vi "DLPVA-100-B_&_F_Set.vi"(6 "Filter":bool=TRUE, 8 "AC/DC":bool=TRUE, 9 "Gain_2 i":bool, 10 "Gain_1 i":bool, 11 "Index":i32) -> (0 "Overload":bool, 1 "Gain_2 o":bool, 2 "Gain_1o":bool, 3 "Gain (dB)":dbl)   [LabVIEW 2013]
uses:
  driver/Control/Set_Bandwidth_DLPVA-Series.vi
  driver/Control/Set_Gain_DLPVA-100-B&F_Series.vi
  driver/FEMTO_LUCI-10.lvlib
panel:
  out "Gain_Stages 2":bool[](array[boolean])=[FALSE, FALSE, FALSE, TRUE, FALSE, FALSE, FALSE, FALSE, FALSE, FALSE, FALSE, FALSE, FALSE, FALSE, FALSE, FALSE, FALSE, FALSE, FALSE, FALSE, FALSE, FALSE, FALSE, FALSE, FALSE, FALSE, FALSE, FALSE, FALSE, FALSE, FALSE, FALSE]
  # "Remote Control LUCI-10 DLPVA-100"
  # "DLPVA-100-B & F"
  # "Configuration"
  # "Gain Setting"
  # "Overal Gain"
  # "80 dB"
  # "60 dB"
  # "Device Information"
  # "40 dB"
  # "20 dB"
  # "Filter"
  # "Coupling"
  # "Sophisticated Tools for Signal Recovery"
  # "AC"
  # "DC"
  # "1 kHz"
  # "100 kHz"
  # "20 dB"
  # "40 dB"
  # "0 dB"
  # "0 dB"
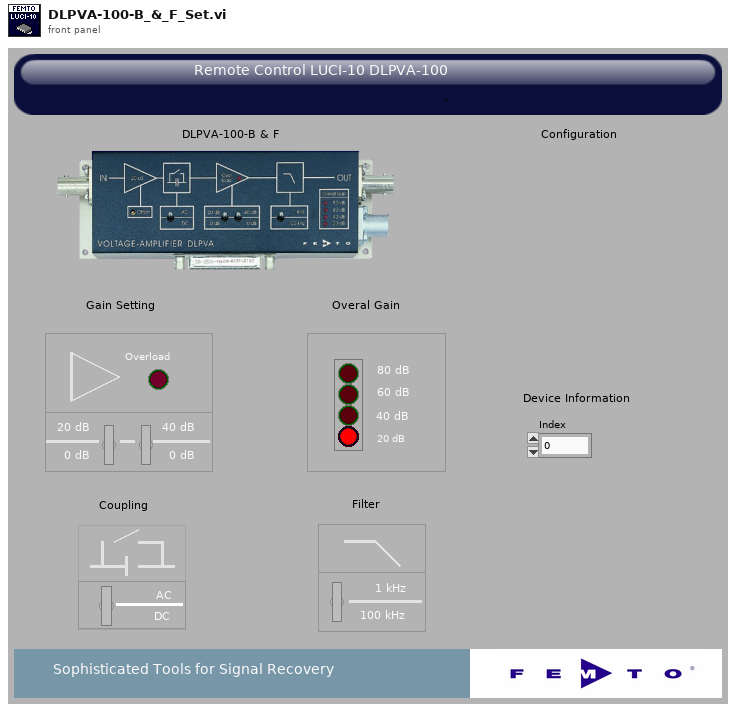
[diagram p1: front panel]
types:
  T1 = enum16{"DDPCA-300", "DLPCA-200", "DHPCA-100", "OE-200", "LIA-MV-150-S", "LIA-MV-150-D", "LIA-MV-200-L", "LIA-MV-200-H", "LIA-MVD-200-L", "LIA-MVD-200-H", "DLPVA-100-BUN-S", "DLPVA-100-BLN-S", "DLPVA-100-B-S", "DLPVA-100-B-D", "DLPVA-100-F-S", "DLPVA-100-F-D", "DHPVA-100", "DHPVA-200", "DUPVA-1-60", "DUPVA-1-70"}
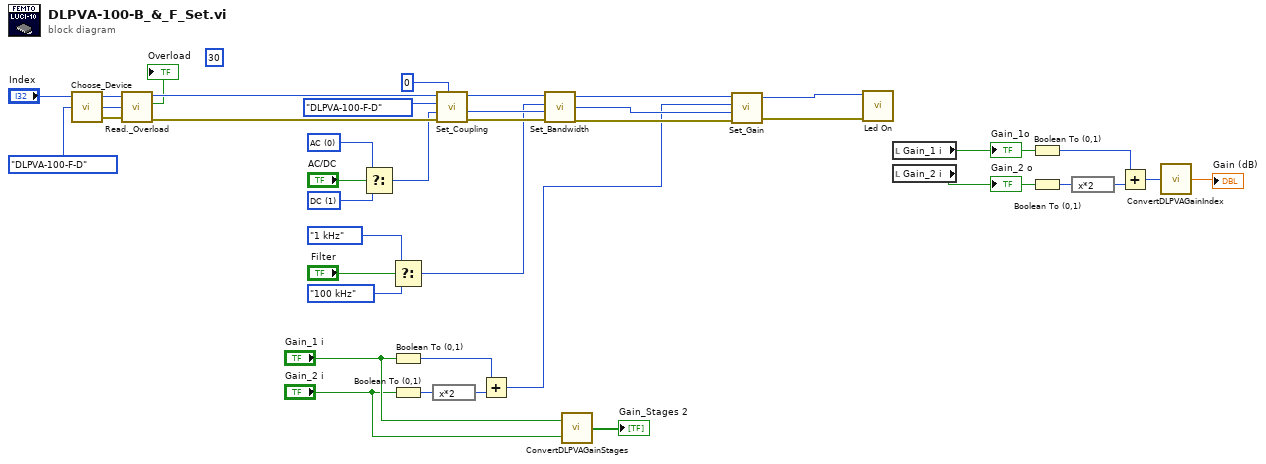
[diagram p0: block diagram]
diagram:
  w11 = u16 1 items=["AC", "DC"] ("Set Coupling")
  w12 = u16 0 items=["AC", "DC"] ("Set Coupling")
  (unwired) 30
  n1 = call "Choose_Device.vi"("Choose_Device"=T1."DLPVA-100-F-D", "Index"="Index") -> ("error out"=w30:errorcluster, "Device_type"=w27:T1, "Index_Out"=w32:i32)  [unwired: 1 in]
  n2 = call "Read._Overload.vi"("Index"=w32, "Choose_Device"=w27, "error in (no error)"=w30) -> ("Index_Out"=w31:i32, "Overload"=→"Overload":bool, "error out"=w29:errorcluster)  [unwired: 1 out]
  n3 = Select(t=w12, s="AC/DC", f=w11) -> (s? t:f=w8:u16)
  n4 = Select(t=enum16{"1 kHz", "100 kHz"}."1 kHz" ("Bandwidth"), s="Filter", f=enum16{"1 kHz", "100 kHz"}."100 kHz" ("Bandwidth")) -> (s? t:f=w18:enum16{"1 kHz", "100 kHz"})
  n5 = Boolean To (0,1)(Boolean="Gain_1 i") -> (0, 1=w6:i16)
  n6 = Boolean To (0,1)(Boolean="Gain_2 i") -> (0, 1=w17:i16)
  n7 = expression code="x*2"(w17) -> (w16:i16)
  n8 = call "Set_Coupling.vi"("Status"=0, "error in (no error)"=w29, "Set Coupling"=w8, "Choose_Device"=T1."DLPVA-100-F-D", "Index"=w31) -> ("error out"=w20:errorcluster, "Status_out"=w21:i32, "Index_Out"=w22:i32)  [unwired: 1 out]
  n9 = Add(x=w6, y=w16) -> (x+y=w7:i16)
  n10 = call-poly "Set_Bandwidth.vi"("error in"=w20, "Status"=w21, "Bandwidth"=w18, "index"=w22) -> ("error out"=w13:errorcluster, "Status_out"=w14:i32, "index_out"=w15:i32)
  n11 = call "ConvertDLPVAGainStages.vi"("Gain_2 i"="Gain_2 i", "Gain_1 i"="Gain_1 i") -> ("Array"=→"Gain_Stages 2":bool[])
  n12 = call-poly "Set_Gain.vi"("error in"=w13, "Status"=w14, "Gain [dB]"=w7, "index"=w15) -> ("error out"=w1:errorcluster, "index_out"=w2:i32)  [unwired: 1 out]
  n13 = call "Led On.vi"("error in (no error)"=w1, "index"=w2) -> ()  [unwired: 7 in, 3 out]
  n14 = local read "Gain_1 i"() -> (w35:bool)
  "Gain_1o" <- w35
  n15 = local read "Gain_2 i"() -> (w34:bool)
  "Gain_2 o" <- w34
  n16 = Boolean To (0,1)(Boolean=w35) -> (0, 1=w40:i16)
  n17 = Boolean To (0,1)(Boolean=w34) -> (0, 1=w38:i16)
  n18 = expression code="x*2"(w38) -> (w39:i16)
  n19 = Add(x=w40, y=w39) -> (x+y=w37:i16)
  n20 = call "ConvertDLPVAGainIndex.vi"("Numeric 2"=w37) -> ("Numeric"=→"Gain (dB)":dbl)
